vi "RT Apply Target Disk Image.vi"(4 "file blacklist":string[](array[string]), 6 "restart after imaging? (T)":bool=TRUE, 8 "error in (no error)":errorcluster, 10 "image file path":path, 11 "target address":string) -> (0 "error out":errorcluster, 3 "IP settings after restart":T1)   [LabVIEW 2020, in "NI_Real-Time Libraries.lvlib"]
doc: "LabVIEW no longer supports this VI. For information about replacing the RT Utility VIs, refer to ni.com/info and enter the Info Code RT_Utility_Replace. Replaces the entire contents of the primary hard drive on the RT target with the files in the target disk image you specify.\n\n<B>target address</B> specifies the IP address or DNS name of the target. \n\n<B>image file path</B> specifies the local path of the disk image to load onto the RT target. \n\n<B>error in</B> describes error conditions that occur before this node runs. This input provides standard error in functionality. \n\n<B>restart after imaging</B> specifies whether to restart the target after applying the target disk image. If this input is FALSE, the RT target remains in install mode after this VI runs. If this input is TRUE, the RT target restarts into normal running mode.\n\n<B>file blacklist</B> specifies an array of file paths to exclude from the target image. To enable filtering through strict matching, the data type of this control is an array of strings rather than an array of paths. \n\n<B>IP settings after restart</B> returns the IP settings of the RT target. If the IP settings change upon restarting, this output returns the new IP settings that take effect after the target restarts. If the previous IP address of the target is in use by another device on the network and the target is configured to use DHCP, the IP address of the target might change upon restarting.\n\n<B>IP address</B> is the IP address of the networked device. \n\n<B>DNS name</B> is the network DNS name of the target. \n\n<B>subnet mask</B> is the bit mask used to identify the subnet in which the target resides on the network. \n\n<B>gateway</B> is the network gateway used by the target. \n\n<B>DNS server</B> is the domain name server used by the target. \n\n<B>error out</B> contains error information. This output provides standard error out functionality. \n\n\nRT Apply Target Disk Image Details\nIf you need to perform additional configuration operations, set <B>restart after imaging?</B> to FALSE. When <B>restart after imaging?</B> is FALSE, <B>IP settings after restart</B> returns an empty cluster. When <B>restart after imaging?</B> is TRUE, this VI waits to finish until the real-time operating system has started and can communicate over the network. However, because the RT target requires additional time to load LabVIEW, drivers, and startup applications, you might need to allow additional time before using the target. To avoid IP conflicts, this VI attempts to preserve the existing IP settings of the target.\n\nThis VI does not support the following use cases. Disk images based on RT targets with multiple operating systems or multiple hard disk partitions. Disk images created using an RT Desktop PC Utility USB drive. Disk images created from a target with a model code different from the model code of the target at <B>target address</B>."
uses:
  <vilib>/real-time/NI_Real-Time Libraries.lvlib
  <vilib>/real-time/rtutility.llb/subVIs/IP Settings.ctl
  <vilib>/zip/NI_Unzip.lvlib
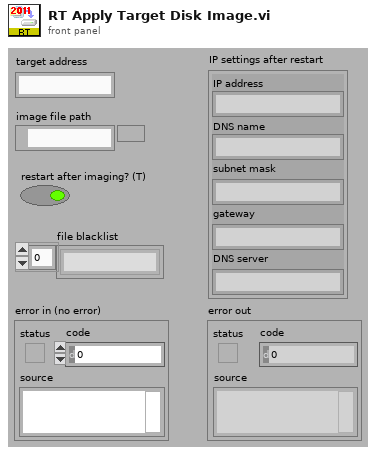
[diagram p1: front panel]
types:
  T1 = typedef "NI_Real-Time Libraries.lvlib/IP Settings.ctl" = cluster{"IP address":string, "DNS name":string, "subnet mask":string, "gateway":string, "DNS server":string}
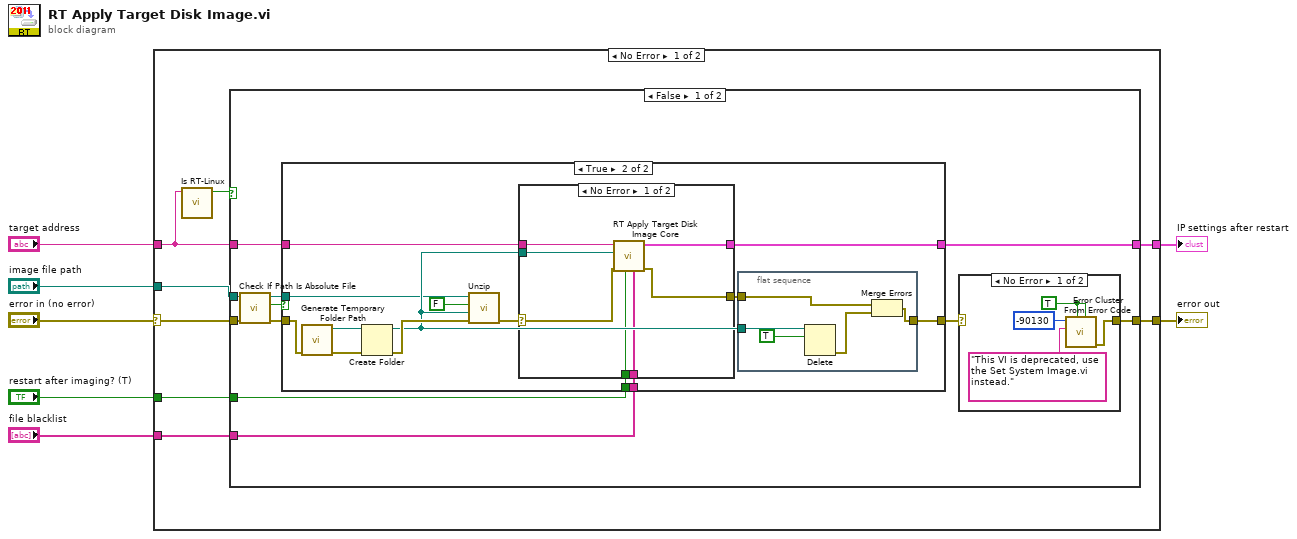
[diagram p0: block diagram]
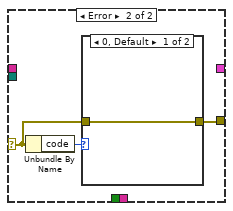
[diagram p4: hidden frame]
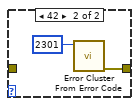
[diagram p5: hidden frame]
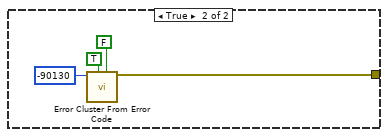
[diagram p6: hidden frame]
diagram:
  n1 = case shown="No Error" "error in (no error)" {
    selector: "error in (no error)" -> [w12 w69]
    tunnel: "target address" -> [w8 _]
    tunnel: "image file path" -> [w11 _]
    tunnel: "restart after imaging? (T)" -> [w15 _]
    tunnel: "file blacklist" -> [w14 _]
    tunnel: [w13 _] -> w3
    tunnel: [w10 w69] -> w2
    frame No Error {
      n2 = call <vilib>:"Is RT-Linux.vi"("target address"=w8) -> ("Is RT-Linux?"=w9:bool)  [unwired: 10 in]
      n3 = case shown="False" w9 {
        tunnel: w8 -> [w26 _]
        tunnel: w15 -> [w25 _]
        tunnel: w14 -> [w24 _]
        tunnel: [w23 _] -> w13
        tunnel: w12 -> [w22 _]
        tunnel: w11 -> [w21 _]
        tunnel: [w16 w68] -> w10
        frame False {
          n4 = call <vilib>:"Check If Path Is Absolute File.vi"("error in (no error)"=w22, "path"=w21) -> ("error out"=w20:errorcluster, "is absolute file?"=w18:bool, "path out"=w19:path)  [unwired: 7 out]
          n5 = case shown="True" w18 {
            tunnel: w26 -> [_ w46]
            tunnel: w25 -> [_ w41]
            tunnel: w24 -> [_ w40]
            tunnel: [_ w39] -> w23
            tunnel: w20 -> [w32 w37]
            tunnel: w19 -> [_ w36]
            tunnel: [w32 w35] -> w17
            frame False {
            }
            frame True {
              n6 = call <vilib>:"Generate Temporary Folder Path.vi"("error in (no error)"=w37) -> ("error out"=w45:errorcluster, "Unique Temporary Folder Path"=w44:path)  [unwired: 9 out]
              n7 = Create Folder(path (use dialog)=w44, error in=w45) -> (created path=w38:path, error out=w42:errorcluster)  [unwired: 1 in, 1 out]
              n8 = call <vilib>:"Unzip.vi"("error in (no error)"=w42, "Target directory (same as Zip file if empty)"=w38, "Preview only?"=FALSE, "Zip file"=w36) -> ("error out"=w33:errorcluster)  [unwired: 7 out]
              n9 = case shown="No Error" w33 {
                selector: w33 -> [w47 w54]
                tunnel: w46 -> [w53 _]
                tunnel: w41 -> [w52 _]
                tunnel: w40 -> [w51 _]
                tunnel: [w50 _] -> w39
                tunnel: w38 -> [w49 _]
                tunnel: [w48 w55] -> w34
                frame No Error {
                  n10 = call <vilib>:"RT Apply Target Disk Image Core.vi"("file blacklist"=w51, "restart after imaging? (T)"=w52, "error in (no error)"=w47, "image path"=w49, "target address"=w53) -> ("error out"=w48:errorcluster, "IP settings after restart"=w50:T1)  [unwired: 5 out]
                }
                frame Error {
                  n11 = Unbundle By Name(w54) -> ("code"=w56:i32)
                  n12 = case shown="0, Default" w56 {
                    tunnel: [w57 w59] -> w55
                    tunnel: w54 -> [w57 _]
                    frame 0, Default {
                    }
                    frame 42 {
                      n13 = call <vilib>:"Error Cluster From Error Code.vi"("error code (0)"=2301) -> ("error out"=w59:errorcluster)  [unwired: 2 in, 6 out]
                    }
                  }
                }
              }
              n14 = flat-sequence {
                tunnel: w38 -> [w64]
                tunnel: w34 -> [w61]
                tunnel: [w60] -> w35
                frame #0 {
                  n15 = Delete(path (use dialog)=w64, entire hierarchy (F)=TRUE) -> (error out=w62:errorcluster)  [unwired: 1 in, 4 out]
                  n16 = Merge Errors(w61, w62) -> (w60:errorcluster)
                }
              }
            }
          }
          n17 = case shown="No Error" w17 {
            selector: w17 -> [_ w31]
            tunnel: [w27 w31] -> w16
            frame No Error {
              w29 = TRUE ("show call chain? (False)")
              n18 = call <vilib>:"Error Cluster From Error Code.vi"("is warning? (False)"=w29, "show call chain? (False)"=w29, "error message (\"\")"="This VI is deprecated, use the Set System Image.vi instead.", "error code (0)"=-90130) -> ("error out"=w27:errorcluster)  [unwired: 5 in]
            }
            frame Error {
            }
          }
        }
        frame True {
          n19 = call <vilib>:"Error Cluster From Error Code.vi"("is warning? (False)"=FALSE, "show call chain? (False)"=TRUE, "error code (0)"=-90130) -> ("error out"=w68:errorcluster)  [unwired: 6 in]
        }
      }
    }
    frame Error {
    }
  }
  "IP settings after restart" <- w3
  "error out" <- w2
